vi "Cache_PPL Global.vi"() -> ()   [LabVIEW 2019, in "ClassLoader.lvlib"]
uses:
  ClassLoader.lvlib
  Ctl/Ctl_PPL Details.ctl
panel:
  in  "PPL Cache Path":map{string, path}(c390)
  in  "PPL Details":map{string, T1}(c390)
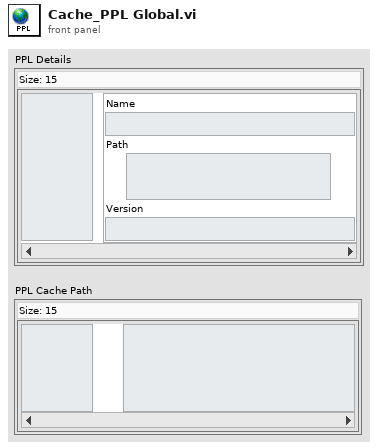
[diagram p1: front panel]
types:
  T1 = typedef "ClassLoader.lvlib/Ctl_PPL Details.ctl" = cluster{"Name":string, "Path":path, "Version":string}
diagram:
